vi "Read Movie Name.vi"(8 "error in (no error)":errorcluster, 11 "Adam Sandler in":refnum<class "Adam Sandler.lvclass">) -> (0 "error out":errorcluster, 2 "Movie Name":string, 3 "Adam Sandler out":refnum<class "Adam Sandler.lvclass">)   [LabVIEW 2019, in "Adam Sandler.lvclass"]
uses:
  Adam Sandler.lvclass
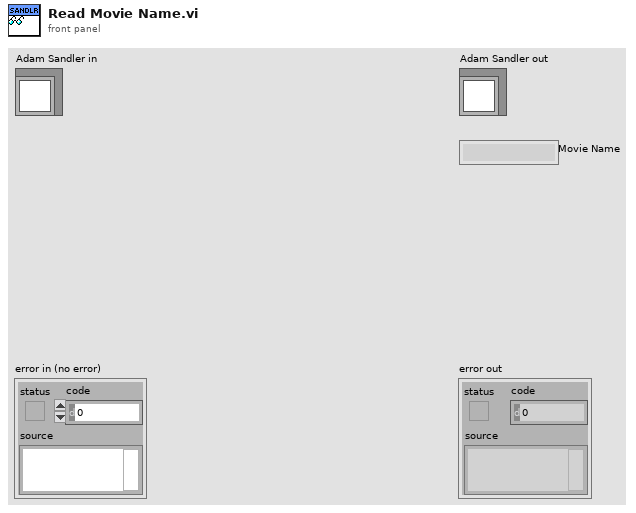
[diagram p1: front panel]
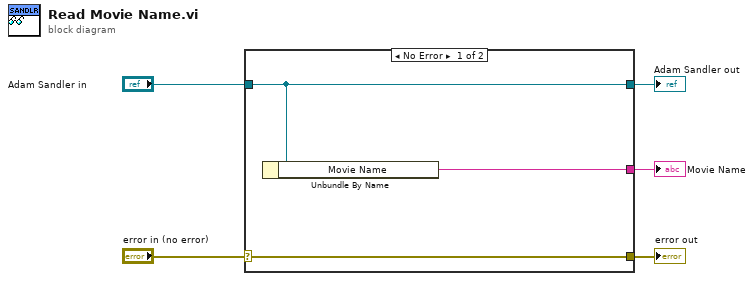
[diagram p0: block diagram]
diagram:
  n1 = case shown="No Error" "error in (no error)" {
    selector: "error in (no error)" -> [w8 w9]
    tunnel: [w8 w9] -> w4
    tunnel: [w7 w10] -> w2
    tunnel: "Adam Sandler in" -> [w7 w10]
    tunnel: [w6 _] -> w1
    frame No Error {
      n2 = Unbundle By Name(w7) -> ("Movie Name"=w6:string)
    }
    frame Error {
    }
  }
  "error out" <- w4
  "Adam Sandler out" <- w2
  "Movie Name" <- w1
